vi "Motor State Toggle.vi"(0 "MotorControlDevRef":T1={"DeviceStatus"={"status"=FALSE, "code"=0, "source"=""}, "Type"=enum."PWM", "PWM"={"Controller"=enum."Controller 1", "PWM Channel"=enum."Invalid", "DeadBand"={"Name"="", "maxPositivePwm"=0, "minPositivePwm"=0, "centerPwm"=0, "maxNegativePwm"=0, "minNegativePwm"=0, "angularRange"=0}}, "CAN"={"Device Number"=0, "Control Mode"=enum."Percent VBus", "Semaphore"=refnum, "Max Vout"=12.0, "TalonSRX Control Mode"=enum."Percent VBus"}, "Invert"=FALSE, "TransformRef"=refnum, "InvTransformRef"=refnum}, 1 "EncoderDevRef":T10={"DevStatus"={"status"=FALSE, "code"=0, "source"=""}, "EncoderIndex"=enum."Invalid", "CounterIndex"=enum."Ctr 1", "DistancePerCount"=2.0, "Decoding Type"=enum."4x"}, 2 "Upper Limit":dbl, 3 "Motor Speed":dbl, 4 "Switch States":bool, 5 "Lower Limit":dbl) -> (15 "At Upper Limit":bool, 18 "At Lower Limit":bool)   [LabVIEW 2014]
uses:
  <vilib>/Rock Robotics/SystemInterfaces/Encoder/FPGA_EncoderIdx.ctl
  <vilib>/Rock Robotics/WPI/Encoder/WPI_EncoderType.ctl
  <vilib>/Rock Robotics/SystemInterfaces/Counter/FPGA_CounterCtrSystemIndex.ctl
  <vilib>/Rock Robotics/WPI/Encoder/WPI_EncoderDevRef.ctl
  <vilib>/Rock Robotics/WPI/PWM/WPI_PWMTransform_ConPane.ctl
  <vilib>/Rock Robotics/WPI/CAN/Jaguar/SubVIs/WPI_CANJaguar_ControlMode.ctl
  <vilib>/Rock Robotics/WPI/CAN/TalonSRX/WPI_CANTalonSRX_APIControlMode.ctl
  <vilib>/Rock Robotics/SystemInterfaces/Typedef/FPGA_TypedefDigitalModule.ctl
  <vilib>/Rock Robotics/SystemInterfaces/DIO/FPGA_DIOPWMChannel.ctl
  <vilib>/Rock Robotics/WPI/PWM/WPI_PWMDeadband.ctl
  <vilib>/Rock Robotics/WPI/MotorControl/WPI_MotorControlType.ctl
  <vilib>/Rock Robotics/WPI/MotorControl/WPI_MotorControlDeviceRef.ctl
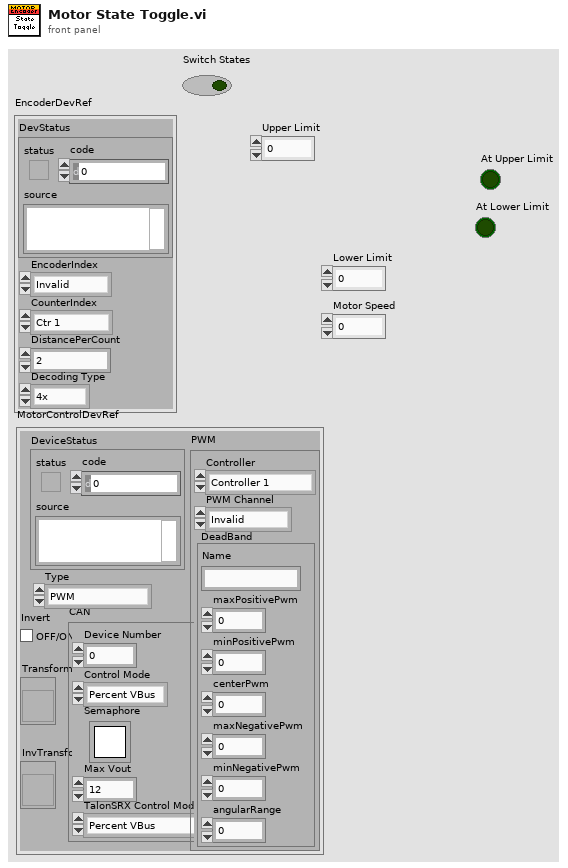
[diagram p1: front panel]
types:
  T1 = typedef "WPI_MotorControlDeviceRef.ctl" = cluster{"DeviceStatus":errorcluster, "Type":T2, "PWM":cluster{"Controller":T3, "PWM Channel":T4, "DeadBand":T5}, "CAN":cluster{"Device Number":u8, "Control Mode":T6, "Semaphore":T7, "Max Vout":dbl, "TalonSRX Control Mode":T8}, "Invert":bool, "TransformRef":T9, "InvTransformRef":T9}
  T2 = typedef "WPI_MotorControlType.ctl" = enum16{"PWM", "CAN", "CANTalonSRX"}
  T3 = typedef "FPGA_TypedefDigitalModule.ctl" = enum16{"Controller 1"}
  T4 = typedef "FPGA_DIOPWMChannel.ctl" = enum8{"PWM 0", "PWM 1", "PWM 2", "PWM 3", "PWM 4", "PWM 5", "PWM 6", "PWM 7", "PWM 8", "PWM 9", "PWM MXP 0", "PWM MXP 1", "PWM MXP 2", "PWM MXP 3", "PWM MXP 4", "PWM MXP 5", "PWM MXP 6", "PWM MXP 7", "PWM MXP 8", "PWM MXP 9", "Invalid"}
  T5 = typedef "WPI_PWMDeadband.ctl" = cluster{"Name":string, "maxPositivePwm":i32, "minPositivePwm":i32, "centerPwm":i32, "maxNegativePwm":i32, "minNegativePwm":i32, "angularRange":u16}
  T6 = typedef "WPI_CANJaguar_ControlMode.ctl" = enum8{"Percent VBus", "Current", "Speed", "Position", "Voltage"}
  T7 = typedef "Semaphore RefNum" = refnum<k1>
  T8 = typedef "WPI_CANTalonSRX_APIControlMode.ctl" = enum8{"Percent VBus", "Speed", "Position", "Slave", "Unchanged / Invalid"}
  T9 = typedef "WPI_PWMTransform_ConPane.ctl" = refnum<vi>
  T10 = typedef "WPI_EncoderDevRef.ctl" = cluster{"DevStatus":errorcluster, "EncoderIndex":T11, "CounterIndex":T12, "DistancePerCount":dbl, "Decoding Type":T13}
  T11 = typedef "FPGA_EncoderIdx.ctl" = enum8{"Enc 0", "Enc 1", "Enc 2", "Enc 3", "Enc 4", "Enc 5", "Enc 6", "Enc 7", "Invalid"}
  T12 = typedef "FPGA_CounterCtrSystemIndex.ctl" = enum8{"Ctr 0", "Ctr 1", "Ctr 2", "Ctr 3", "Ctr 4", "Ctr 5", "Ctr 6", "Ctr 7", "Invalid"}
  T13 = typedef "WPI_EncoderType.ctl" = enum16{"1x", "2x", "4x"}
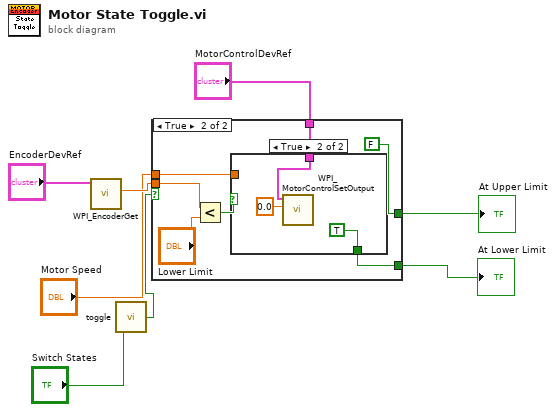
[diagram p0: block diagram]
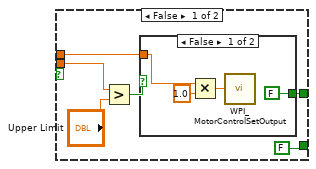
[diagram p2: hidden frame]
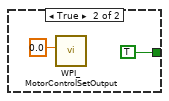
[diagram p3: hidden frame]
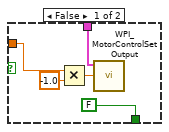
[diagram p4: hidden frame]
diagram:
  n1 = call <vilib>:"WPI_EncoderGet.vi"("EncoderDevRef"="EncoderDevRef") -> ("Distance"=w8:dbl)  [unwired: 5 in, 5 out]
  n2 = call "toggle.vi"("Input"="Switch States") -> ("Output"=w4:bool)
  n3 = case shown="True" w4 {
    tunnel: w8 -> [w12 w26]
    tunnel: "Motor Speed" -> [w11 w24]
    tunnel: "MotorControlDevRef" -> [_ w23]
    tunnel: [w10 FALSE] -> w2
    tunnel: [FALSE ("At Lower Limit") w21] -> w1
    frame False {
      n4 = Greater?(x=w12, y="Upper Limit") -> (0:w13:bool)
      n5 = case shown="False" w13 {
        tunnel: w11 -> [w16 _]
        tunnel: [FALSE TRUE] -> w10
        frame False {
          n6 = Multiply(x=w16, y=1.0) -> (x*y=w17:dbl)
          n7 = call <vilib>:"WPI_MotorControlSetOutput.vi"("Output"=w17) -> ()  [unwired: 8 in, 3 out]
        }
        frame True {
          n8 = call <vilib>:"WPI_MotorControlSetOutput.vi"("Output"=0.0) -> ()  [unwired: 8 in, 3 out]
        }
      }
    }
    frame True {
      n9 = Less?(x=w26, y="Lower Limit") -> (x < y?=w25:bool)
      n10 = case shown="True" w25 {
        tunnel: w24 -> [w30 _]
        tunnel: w23 -> [w29 w34]
        tunnel: [FALSE ("At Lower Limit") TRUE] -> w21
        frame False {
          n11 = Multiply(x=w30, y=-1.0) -> (x*y=w31:dbl)
          n12 = call <vilib>:"WPI_MotorControlSetOutput.vi"("Output"=w31, "MotorControlDevRef"=w29) -> ()  [unwired: 7 in, 3 out]
        }
        frame True {
          n13 = call <vilib>:"WPI_MotorControlSetOutput.vi"("Output"=0.0, "MotorControlDevRef"=w34) -> ()  [unwired: 7 in, 3 out]
        }
      }
    }
  }
  "At Lower Limit" <- w1
  "At Upper Limit" <- w2
